vi "Convertion Ms en Texte.vi"(1 "Numérique":dbl) -> (0 "Chaîne":string)   [LabVIEW 2020, in "Library Commun.lvlib"]
uses:
  Library Commun.lvlib
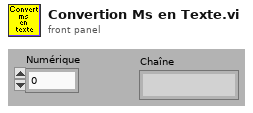
[diagram p1: front panel]
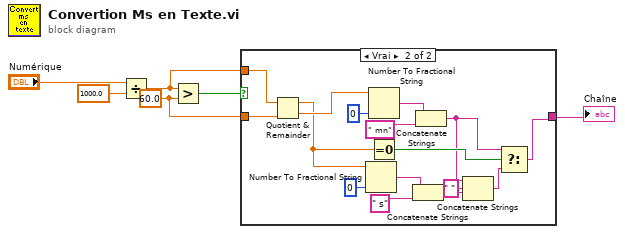
[diagram p0: block diagram]
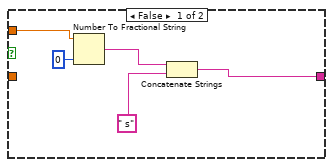
[diagram p2: hidden frame]
diagram:
  w4 = 60.0 ("y")
  n1 = Divide(x="Numérique", y=1000.0) -> (x/y=w3:dbl)
  n2 = Greater?(x=w3, y=w4) -> (0:w5:bool)
  n3 = case shown="Vrai" w5 {
    tunnel: w3 -> [w9 w27]
    tunnel: w4 -> [_ w26]
    tunnel: [w7 w12] -> w6
    frame False {
      n4 = Number To Fractional String(number=w9, precision (6)=i16 0 ("précision (6)")) -> (F-format string=w8:string)  [unwired: 2 in]
      n5 = Concatenate Strings(w8, " s" ("chaîne")) -> (w7:string)
    }
    frame True {
      n6 = Quotient & Remainder(x=w27, y=w26) -> (x-y*floor(x/y)=w18:dbl, floor(x/y)=w24:dbl)
      n7 = Number To Fractional String(number=w18, precision (6)=i16 0 ("précision (6)")) -> (F-format string=w20:string)  [unwired: 2 in]
      n8 = Number To Fractional String(number=w24, precision (6)=i16 0 ("précision (6)")) -> (F-format string=w23:string)  [unwired: 2 in]
      n9 = Equal To 0?(x=w18) -> (x = 0?=w17:bool)
      n10 = Concatenate Strings(w20, " s" ("chaîne")) -> (w15:string)
      n11 = Concatenate Strings(w23, " mn" ("chaîne")) -> (w13:string)
      n12 = Concatenate Strings(w13, " " ("chaîne"), w15) -> (w14:string)
      n13 = Select(t=w13, s=w17, f=w14) -> (s? t:f=w12:string)
    }
  }
  "Chaîne" <- w6
